vi "Dual_SVPWM_TimingGen_SGL_src.vi"(0 "ref_alpha":sgl[](array[numeric])=[0.0, 0.0], 1 "ref_max":sgl=0.9999695, 2 "Period":i32=1, 5 "ref_beta":sgl[](array[numeric])=[0.0, 0.0]) -> (4 "A_timing":T1[](array[typedef]), 6 "B_timing":T1[](array[typedef]), 8 "C_timing":T1[](array[typedef]))   [LabVIEW 2017]
uses:
  SVPWM/ON_OFF_timing.ctl
  SVPWM/SVPWM.lvlib
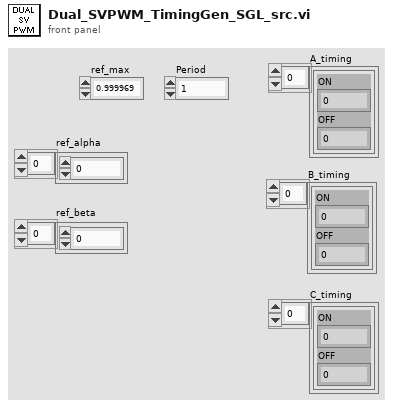
[diagram p1: front panel]
types:
  T1 = typedef "SVPWM.lvlib/ON_OFF_timing.ctl" = cluster{"ON":u32, "OFF":u32}
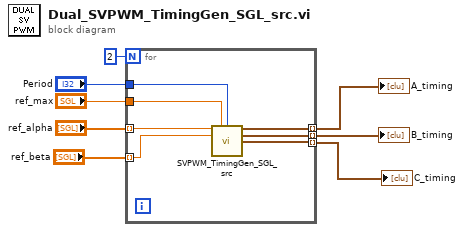
[diagram p0: block diagram]
diagram:
  n1 = for {
    N: 2 -> [_]
    tunnel: "ref_max" -> [w15]
    tunnel: "Period" -> [w14]
    tunnel: [w13] -> w3 mode=indexing
    tunnel: [w12] -> w2 mode=indexing
    tunnel: [w11] -> w1 mode=indexing
    tunnel: "ref_alpha" -> [w10] mode=indexing
    tunnel: "ref_beta" -> [w9] mode=indexing
    n2 = call "SVPWM_TimingGen_SGL_src.vi"("ref_alpha"=w10, "ref_max"=w15, "Period"=w14, "ref_beta"=w9) -> ("A_timing"=w13:T1, "B_timing"=w12:T1, "C_Timing"=w11:T1)  [unwired: 8 in, 1 out]
  }
  "A_timing" <- w3
  "B_timing" <- w2
  "C_timing" <- w1
